vi "niRFUtil RFHS FIFO Create.vi"(0 "Name":string, 1 "Flush":bool=TRUE, 5 "Buffer Size (bytes)":u32=3072000, 11 "error in (no error)":errorcluster) -> (4 "FIFO":T1, 15 "error out":errorcluster)   [LabVIEW 2015, in "niRFUtil.lvlib"]
uses:
  niRFUtil.lvlib
  niRFUtil RFHS FIFO Reference.ctl
  niRFUtil RFHS FIFO.ctl
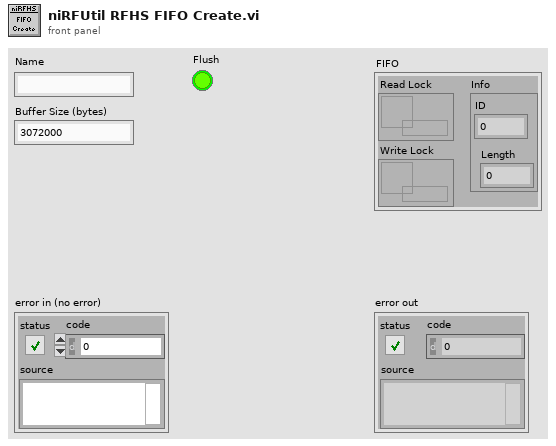
[diagram p1: front panel]
types:
  T1 = typedef "niRFUtil.lvlib/niRFUtil RFHS FIFO Reference.ctl" = cluster{"Read Lock":refnum<data-value>, "Info":T2, "Write Lock":refnum<data-value>}
  T2 = typedef "niRFUtil.lvlib/niRFUtil RFHS FIFO.ctl" = cluster{"ID":u64, "Length":u32}
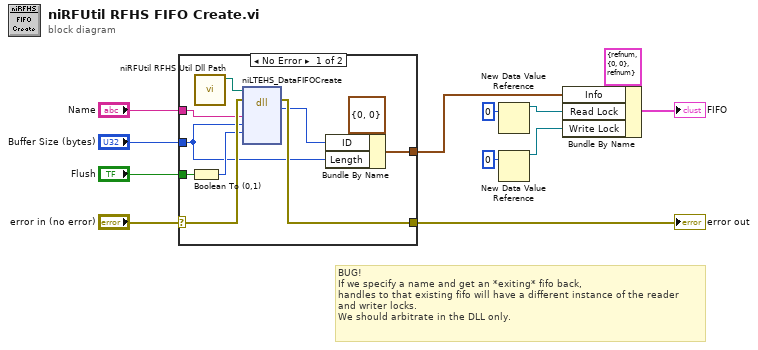
[diagram p0: block diagram]
diagram:
  # "BUG! \nIf we specify a name and get an *exiting* fifo back,\nhandles to that existing fifo will have a different instance of the reader\nand writer locks.\nWe should arbitrate in the DLL only."
  n1 = case shown="No Error" "error in (no error)" {
    selector: "error in (no error)" -> [w21 w23]
    tunnel: [w22 w23] -> w11
    tunnel: "Name" -> [w20 _]
    tunnel: "Buffer Size (bytes)" -> [w13 _]
    tunnel: [w17 _] -> w4
    tunnel: "Flush" -> [w15 _]
    frame No Error {
      n2 = Boolean To (0,1)(Boolean=w15) -> (0, 1=w14:i16)
      n3 = call "niRFUtil RFHS Util Dll Path.vi"() -> ("Path"=w16:path)  [unwired: 7 in, 4 out]
      n4 = dll-call lib="M:/RfProtocols/RFmx/DLLs/niRFHS/trunk/2.0/dist/win32U/niRFHS_avx.dll" fn="niLTEHS_DataFIFOCreate"(path in=w16, error in=w21, "name"=w20, "bufferSize"=w13, "flags"=w14) -> (error out=w22:errorcluster, "return type"=w18:u64)  [unwired: 6 in, 1 out]
      n5 = Bundle By Name(cluster=T2 {"ID"=0, "Length"=0} ("Fifo ID"), "ID"=w18, "Length"=w13) -> (w17:T2)
    }
    frame Error {
    }
  }
  "error out" <- w11
  n6 = New Data Value Reference(data value=0) -> (data value reference=w6:refnum<data-value>)  [unwired: 1 in, 1 out]
  n7 = New Data Value Reference(data value=0) -> (data value reference=w2:refnum<data-value>)  [unwired: 1 in, 1 out]
  n8 = Bundle By Name(cluster=T1 {"Read Lock"=refnum, "Info"={"ID"=0, "Length"=0}, "Write Lock"=refnum} ("FIFO"), "Info"=w4, "Read Lock"=w6, "Write Lock"=w2) -> (→"FIFO":T1)
